vi "TTA_MATLAB_Set_Relay_Mode.vi"(8 "error in":errorcluster, 11 "Mode":T1(ring)) -> (0 "error out":errorcluster, 3 "Success":bool)   [LabVIEW 2016]
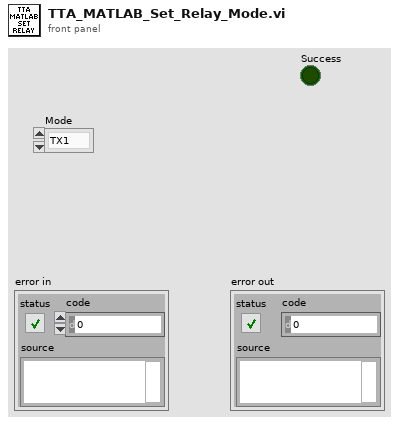
[diagram p1: front panel]
types:
  T1 = enum16{"TX1", "TX2", "TX3", "TX4", "TXx3", "TXx4", "RX1", "RX2", "RX3", "RX4", "RXx3", "RXx4", "RFCal"}
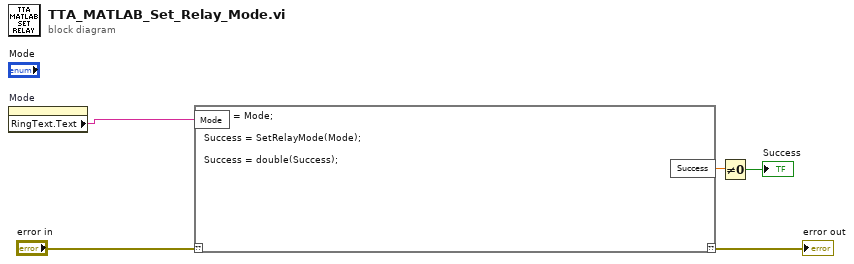
[diagram p0: block diagram]
diagram:
  n1 = property on="Mode" class="Enum (strict)"() -> ("RingText.Text"=w3:string)  [unwired: 2 in, 2 out]
  n2 = script code="Mode = Mode;\n\nSuccess = SetRelayMode(Mode);\n\nSuccess = double(Success);"("??"="error in", "Mode"=w3) -> ("??"=→"error out":errorcluster, "Success"=w2:dbl)
  n3 = Not Equal To 0?(x=w2) -> (x != 0?=→"Success":bool)
